vi "ReleaseBuffer.vi"(8 "error in (no error)":errorcluster, 10 "Pointer and BufferSize":u64[](array[numeric])) -> (0 "error out":errorcluster)   [LabVIEW 2020]
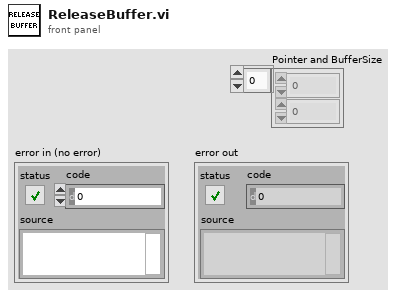
[diagram p1: front panel]
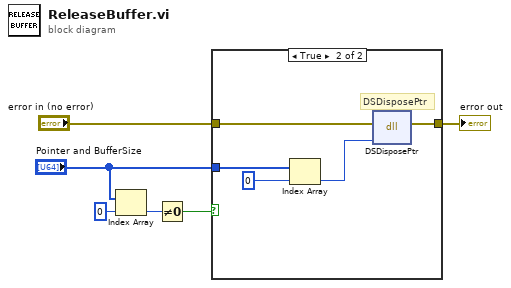
[diagram p0: block diagram]
diagram:
  n1 = Index Array(array="Pointer and BufferSize", index=0) -> (element=w2:u64)
  n2 = Not Equal To 0?(x=w2) -> (x != 0?=w1:bool)
  n3 = case shown="True" w1 {
    tunnel: [w7 w12] -> w6
    tunnel: "error in (no error)" -> [w7 w11]
    tunnel: "Pointer and BufferSize" -> [_ w8]
    frame False {
    }
    frame True {
      # "DSDisposePtr"
      n4 = Index Array(array=w8, index=0) -> (element=w10:u64)
      n5 = dll-call lib="LabVIEW" fn="DSDisposePtr"(error in=w11, "Pointer"=w10) -> (error out=w12:errorcluster)  [unwired: 4 in, 1 out]
    }
  }
  "error out" <- w6
